vi "ROTPEN Model Validation.vi"() -> ()   [LabVIEW 2018]
uses:
  <vilib>/Simulation/Implementation/XNodeFramework/SimXNode/SimX.xnode
  <vilib>/Simulation/Scripting/Companion Diagram/SimConfigNode/SimDog.xnode
  <vilib>/Simulation/SignalArithmetic/Implementation/NILVSim Gain.llb/SIM Gain (scalar).vi
  <vilib>/Quanser/Rapid Control Prototyping Toolkit/hardware/HIL Immediate IO/CL HIL Read.vi
  <vilib>/Simulation/Implementation/Shared/SIMSCR Execution Mode.ctl
  <vilib>/Simulation/Scripting/Companion Diagram/SimConfigNode/_simSolvers.ctl
  <vilib>/Simulation/Scripting/Companion Diagram/SimConfigNode/SimParams.ctl
  <vilib>/Simulation/Utility/Implementation/SIM Halt.vi
  <vilib>/Quanser/Rapid Control Prototyping Toolkit/hardware/HIL Immediate IO/_TypeSpecific/CL HIL Read Encoder (Vector).vi
  <vilib>/Simulation/ContinuousLinear/Implementation/NILVSim Derivative.llb/SIM derivative (scalar).vi
  <vilib>/Simulation/ContinuousLinear/Implementation/NILVSim Transfer Function.llb/SIM Transfer Function (SISO).vi
panel:
  out "Hub Angle (deg)":dbl(graph)
  in  "stop":bool
  out "Pendulum Angle (deg)":dbl(graph)
  # "Rotary Hub Angle:  Deg"
  # "Pendulum Angle:  Deg"
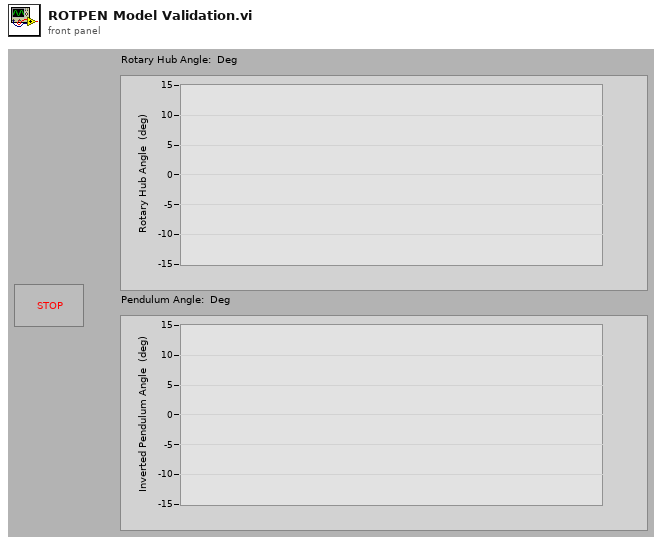
[diagram p1: front panel]
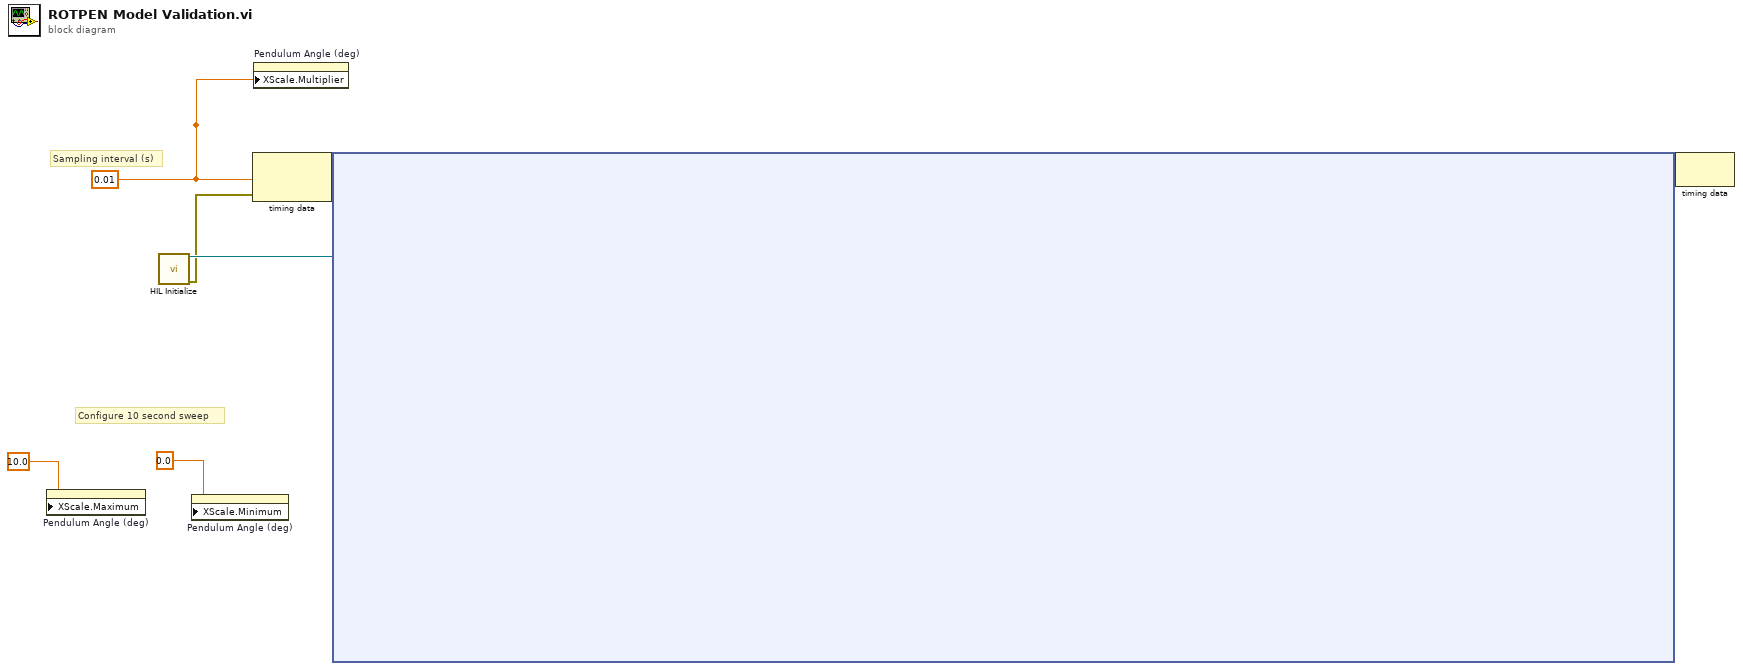
[diagram p0: block diagram]
diagram:
  w3 = 0.01 ("Step Size (s)")
  # "Configure 10 second sweep"
  # "Sampling interval (s)"
  n1 = property on="Pendulum Angle (deg)" class="WFChart (strict)"("XScale.Maximum"=10.0 ("X Scale.Range:Maximum")) -> ()  [unwired: 2 in, 2 out]
  n2 = call "HIL Initialize"() -> ("board out"=w5:refnum<class "HIL Board.lvclass">, "error out"=w4:errorcluster)  [unwired: 14 in]
  n3 = property on="Pendulum Angle (deg)" class="WFChart (strict)"("XScale.Minimum"=0.0 ("X Scale.Range:Maximum")) -> ()  [unwired: 2 in, 2 out]
  n4 = node-c288(w3, w4) -> (w7:variant)
  n5 = property on="Pendulum Angle (deg)" class="WFChart (strict)"("XScale.Multiplier"=w3) -> ()  [unwired: 2 in, 2 out]
  n6 = node-c254 ("Control & Simulation Loop")(w7, w5) -> (w6:variant)
  n7 = node-c288(w6) -> ()  [unwired: 1 out]
